vi "SUB_VolMeasure.vi"(1 "Channel":string, 2 "samples per channel":i32=200, 3 "input terminal configuration":i32(ring)=10083 items=["default"=-1, "RSE"=10083, "NRSE"=10078, "Differential"=10106, "Pseudodifferential"=12529], 4 "Checkversion":u16(ring) items=["Run", "Check Version"]) -> (5 "AVG_Vol":dbl format="%.5f", 6 "Version":string="VolMeasure_0.0.2")   [LabVIEW 2011]
uses:
  <vilib>/DAQmx/read.llb/DAQmx Read (Analog 1D DBL 1Chan NSamp).vi
  <vilib>/DAQmx/create/channels.llb/DAQmx Create Channel (AI-Voltage-Basic).vi
  <vilib>/DAQmx/configure/timing.llb/DAQmx Timing (Sample Clock).vi
  <vilib>/DAQmx/miscellaneous.llb/DAQmx Fill In Error Info.vi
  <vilib>/Analysis/NI_AALBase.lvlib
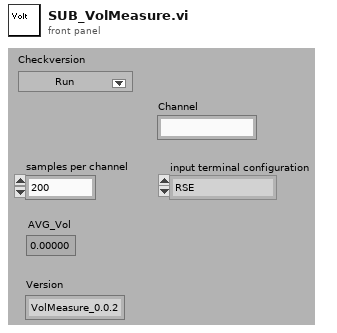
[diagram p1: front panel]
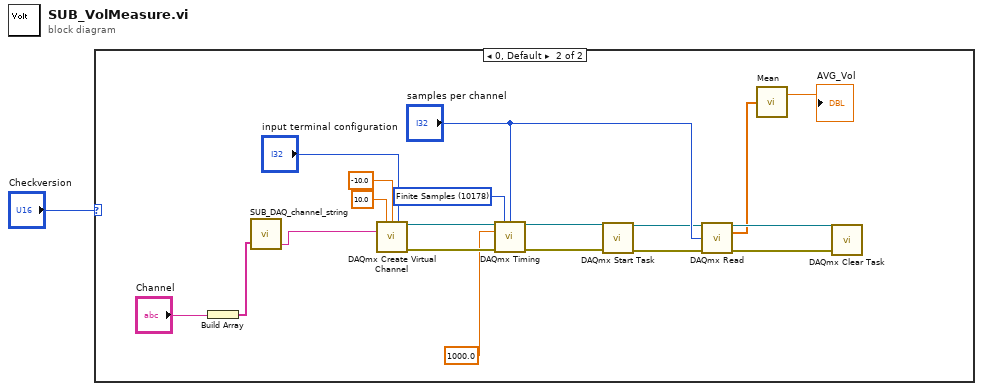
[diagram p0: block diagram]
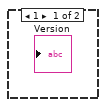
[diagram p2: hidden frame]
diagram:
  n1 = case shown="0, Default" "Checkversion" {
    frame 1 {
    }
    frame 0, Default {
      w17 = 10178 items=["Finite Samples"=10178, "Continuous Samples"=10123, "Hardware Timed Single Point"=12522] ("sample mode")
      n2 = Build Array("Channel") -> (w2:string[])
      n3 = call "SUB_DAQ_channel_string.vi"("channel"=w2) -> ("resulting string"=w4:string)  [unwired: 1 in, 2 out]
      n4 = call-poly <vilib>:"DAQmx Create Virtual Channel.vi"("maximum value"=10.0, "minimum value"=-10.0, "input terminal configuration"="input terminal configuration", "physical channels"=w4) -> ("task out"=w6:refnum<k21>, "error out"=w18:errorcluster)  [unwired: 10 in]
      n5 = call-poly <vilib>:"DAQmx Timing.vi"("task/channels in"=w6, "sample mode"=w17, "samples per channel"="samples per channel", "rate"=1000.0, "error in"=w18) -> ("task out"=w15:refnum<k21>, "error out"=w14:errorcluster)  [unwired: 9 in]
      n6 = call <vilib>:"DAQmx Start Task.vi"("task/channels in"=w15, "error in"=w14) -> ("task out"=w5:refnum<k21>, "error out"=w13:errorcluster)  [unwired: 12 in]
      n7 = call-poly <vilib>:"DAQmx Read.vi"("task/channels in"=w5, "number of samples per channel"="samples per channel", "error in"=w13) -> ("task out"=w11:refnum<k21>, "data"=w9:dbl[], "error out"=w10:errorcluster)  [unwired: 10 in]
      n8 = call <vilib>:"Mean.vi"("X"=w9) -> ("mean"=→"AVG_Vol":dbl)  [unwired: 1 out]
      n9 = call <vilib>:"DAQmx Clear Task.vi"("task in"=w11, "error in"=w10) -> ()  [unwired: 13 in, 1 out]
    }
  }
